vi "Create-Reset 0 SGL Image.vi"(8 "Error In":errorcluster, 9 "Image Characteristics":T2 {"Calibration"."Y Step" format="%.2f"; "Calibration"."X Step" format="%.2f"; "Image Type" items=["Grayscale (U8)", "Grayscale (I16)", "Grayscale (SGL)", "Complex (CSG)", "RGB (U32)", "HSL (U32)", "RGB (U64)", "Grayscale (U16)"]}, 10 "Image Name":string="Image Sum", 11 "Image":T1) -> (0 "Error Out":errorcluster, 3 "New Image":T1)   [LabVIEW 2021, in "Image.lvlib"]
uses:
  Image Characteristics.ctl
  <vilib>/vision/Image Controls.llb/IMAQ Image.ctl
  Image.lvlib
  <vilib>/vision/NI_Vision_Development_Module.lvlib
  Error/Error.lvlib
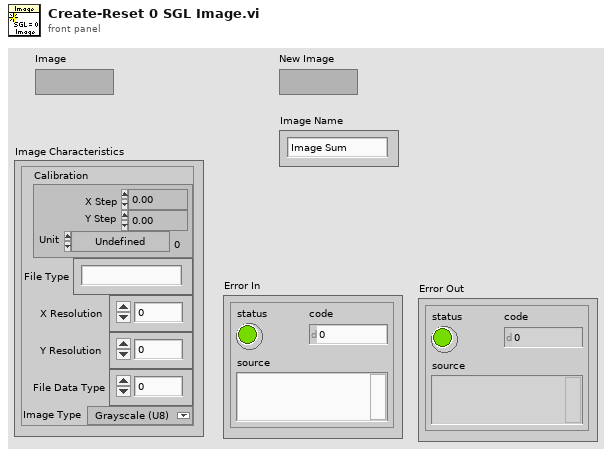
[diagram p1: front panel]
types:
  T1 = typedef "IMAQ Image.ctl" = refnum<image>
  T2 = typedef "Image.lvlib/Image Characteristics.ctl" = cluster{"Calibration":T3, "File Type":string, "X Resolution":i32, "Y Resolution":i32, "File Data Type":i32, "Image Type":T5}
  T3 = typedef "Simple Grid Descriptor" = cluster{"X Step":sgl, "Y Step":sgl, "Unit":T4}
  T4 = typedef "Image Unit" = enum32{"Undefined", "Angström", "Micrometer", "Millimeter", "Centimeter", "Meter", "Kilometer", "Microinch", "Inch", "Feet", "Nautical miles", "Standard miles", "Steps"}
  T5 = typedef "Image Type" = u32
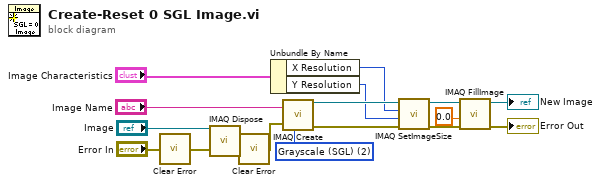
[diagram p0: block diagram]
diagram:
  w6 = T5 2 items=["Grayscale (U8)", "Grayscale (I16)", "Grayscale (SGL)", "Complex (CSG)", "RGB (U32)", "HSL (U32)", "RGB (U64)", "Grayscale (U16)"] ("Image Type")
  n1 = call "Clear Error.vi"("Error In"="Error In") -> ("no Error Out"=w1:errorcluster)  [unwired: 8 in]
  n2 = call "IMAQ Dispose"("Image"="Image", "error in (no error)"=w1) -> ("error out"=w3:errorcluster)  [unwired: 4 in]
  n3 = call "Clear Error.vi"("Error In"=w3) -> ("no Error Out"=w2:errorcluster)  [unwired: 8 in]
  n4 = Unbundle By Name("Image Characteristics") -> ("X Resolution"=w5:i32, "Y Resolution"=w4:i32)
  n5 = call "IMAQ Create"("Image Name"="Image Name", "Image Type"=w6, "error in (no error)"=w2) -> ("New Image"=w15:T1, "error out"=w16:errorcluster)  [unwired: 2 in]
  n6 = call "IMAQ SetImageSize"("error in (no error)"=w16, "Y Resolution"=w4, "X Resolution"=w5, "Image"=w15) -> ("error out"=w13:errorcluster, "Image Out"=w14:T1)  [unwired: 1 in]
  n7 = call "IMAQ FillImage"("error in (no error)"=w13, "Pixel Value (U8, U16, I16, Float)"=sgl 0.0, "Image"=w14) -> ("error out"=→"Error Out":errorcluster, "Image Out"=→"New Image":T1)  [unwired: 7 in]
